vi "Step Add CONT W Parameters.vi"(0 "VISA resource name":refnum<visa-resource-name>, 1 "Continuity Test Paramameters":T2={"High Limit (0 - 10,000 ohms) (1000)"=1000.0, "Low Limit (0 - 10,000 ohms) (0)"=0.0, "Dwell Time (0.0, 0.4 - 999.9 seconds) (1.0)"=1.0, "Offset (0 - 10.00 ohms) (0)"=0.0, "Auto Offset (F: Off)"=FALSE} {"Offset (0 - 10.00 ohms) (0)" format="%.2f"; "Dwell Time (0.0, 0.4 - 999.9 seconds) (1.0)" format="%.1f"; "Low Limit (0 - 10,000 ohms) (0)" format="%.2f"; "High Limit (0 - 10,000 ohms) (1000)" format="%.2f"}, 2 "Internal Scanner Exists?":bool, 3 "Scanner Settings":T1={"Scan1"=1, "Scan2"=1, "Scan3"=1, "Scan4"=1, "Scan5"=1, "Scan6"=1, "Scan7"=1, "Scan8"=1, "Scan9"=1, "Scan10"=1, "Scan11"=1, "Scan12"=1, "Scan13"=1, "Scan14"=1, "Scan15"=1, "Scan16"=1} {"Scan16" scale=0.0..2.0; "Scan15" scale=0.0..2.0; "Scan14" scale=0.0..2.0; "Scan13" scale=0.0..2.0; "Scan12" scale=0.0..2.0; "Scan11" scale=0.0..2.0; "Scan10" scale=0.0..2.0; "Scan9" scale=0.0..2.0; "Scan8" scale=0.0..2.0; "Scan7" scale=0.0..2.0; "Scan6" scale=0.0..2.0; "Scan5" scale=0.0..2.0; "Scan4" scale=0.0..2.0; "Scan3" min=0 max=2 scale=0.0..2.0; "Scan2" min=0 max=2 scale=0.0..2.0; "Scan1" min=0 max=2 scale=0.0..2.0}, 7 "Step Selection (1-200)":i32=1, 9 "Add Step":bool, 11 "error in (no error)":errorcluster) -> (4 "VISA resource name out":refnum<visa-resource-name>, 15 "error out":errorcluster)   [LabVIEW 2012, in "Associated Research 78XX Series.lvlib"]
doc: "Sets the parameters for the CONT test mode for the given memory location."
uses:
  <instrlib>/Associated Research 78XX Series/Associated Research 78XX Series.lvlib
  <instrlib>/Associated Research 78XX Series/Public/Configure/Steps/Low Level/CONT Test Parameters.ctl
  <instrlib>/Associated Research 78XX Series/Public/Configure/Steps/Low Level/Scanner Settings.ctl
panel:
  # "Add"
  # "Edit"
  # "On\nOff"
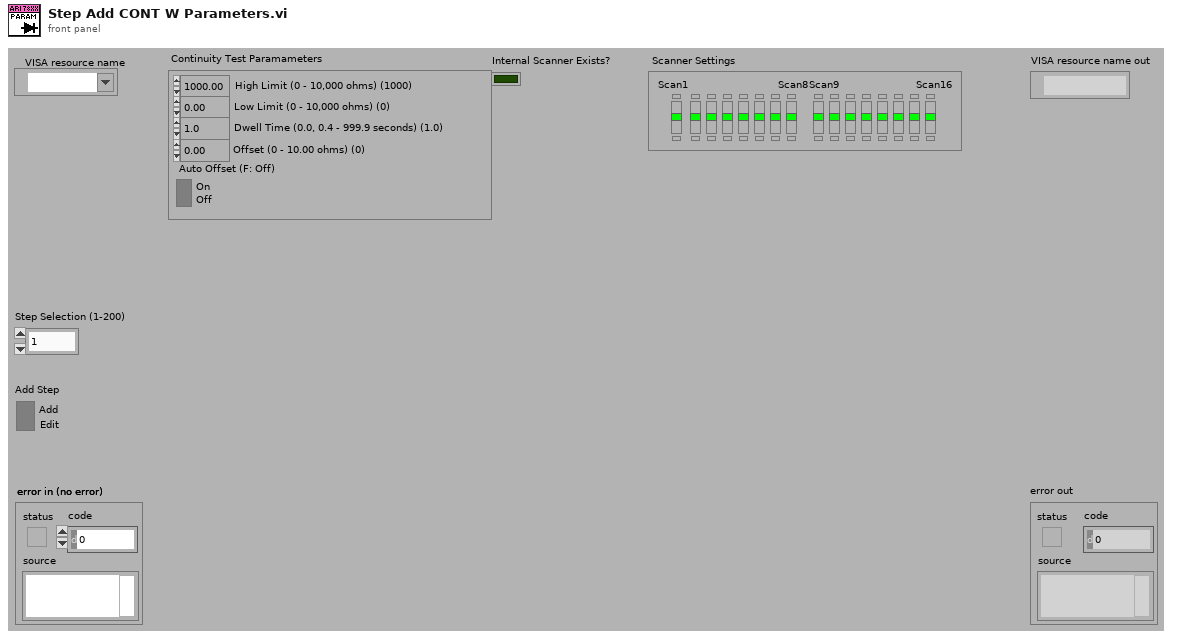
[diagram p1: front panel]
types:
  T1 = typedef "Associated Research 78XX Series.lvlib/Scanner Settings.ctl" = cluster{"Scan1":i32, "Scan2":i32, "Scan3":i32, "Scan4":i32, "Scan5":i32, "Scan6":i32, "Scan7":i32, "Scan8":i32, "Scan9":i32, "Scan10":i32, "Scan11":i32, "Scan12":i32, "Scan13":i32, "Scan14":i32, "Scan15":i32, "Scan16":i32}
  T2 = typedef "Associated Research 78XX Series.lvlib/CONT Test Parameters.ctl" = cluster{"High Limit (0 - 10,000 ohms) (1000)":dbl, "Low Limit (0 - 10,000 ohms) (0)":dbl, "Dwell Time (0.0, 0.4 - 999.9 seconds) (1.0)":dbl, "Offset (0 - 10.00 ohms) (0)":dbl, "Auto Offset (F: Off)":bool}
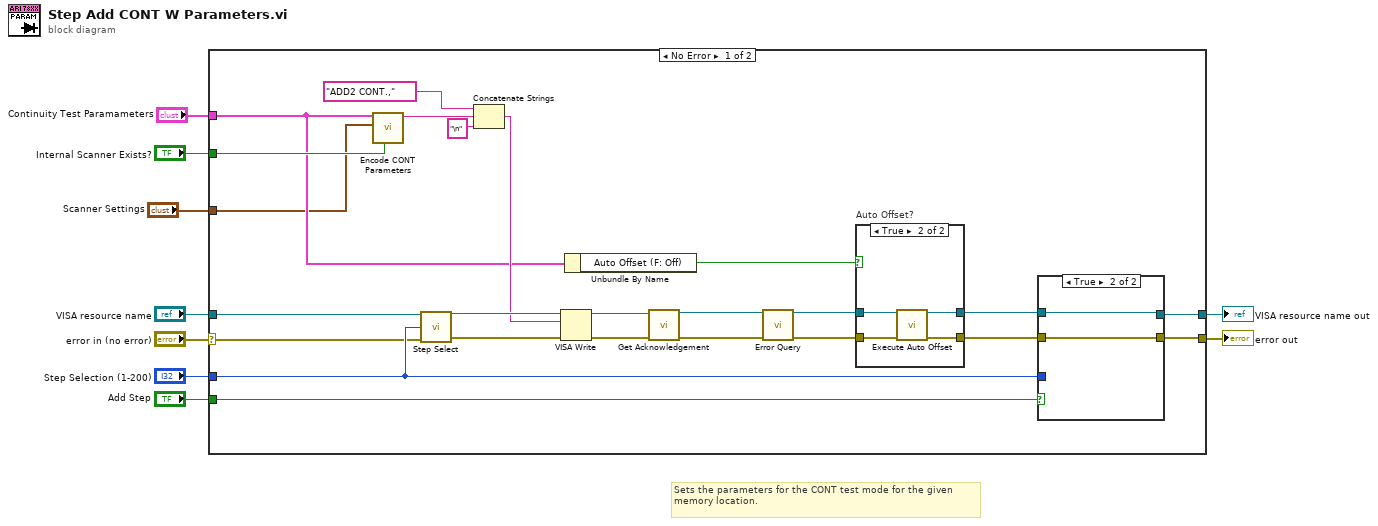
[diagram p0: block diagram]
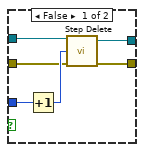
[diagram p3: hidden frame]
diagram:
  # "Sets the parameters for the CONT test mode for the given memory location."
  n1 = case shown="No Error" "error in (no error)" {
    selector: "error in (no error)" -> [w12 w49]
    tunnel: [w31 w49] -> w8
    tunnel: [w30 w48] -> w6
    tunnel: "VISA resource name" -> [w13 w48]
    tunnel: "Step Selection (1-200)" -> [w14 _]
    tunnel: "Add Step" -> [w29 _]
    tunnel: "Continuity Test Paramameters" -> [w16 _]
    tunnel: "Internal Scanner Exists?" -> [w28 _]
    tunnel: "Scanner Settings" -> [w15 _]
    frame No Error {
      n2 = call <instrlib>:"Encode CONT Parameters.vi"("Internal Scanner Exists?"=w28, "Scanner Settings"=w15, "Continuity Test Paramameters in"=w16) -> ("Add Step"=w27:string)  [unwired: 6 in, 2 out]
      n3 = call <instrlib>:"Step Select.vi"("VISA resource name"=w13, "Step Number (1)"=w14, "error in (no error)"=w12) -> ("VISA resource name out"=w32:refnum<visa-resource-name>, "error out"=w33:errorcluster)  [unwired: 11 in]
      n4 = Concatenate Strings("ADD2 CONT.," ("string"), w27, "\n" ("string")) -> (w25:string)
      n5 = VISA Write(VISA resource name=w32, write buffer=w25, error in (no error)=w33) -> (VISA resource name out=w11:refnum<visa-resource-name>, error out=w10:errorcluster)  [unwired: 1 out]
      n6 = Unbundle By Name(w16) -> ("Auto Offset (F: Off)"=w20:bool)
      n7 = call <instrlib>:"Get Acknowledgement.vi"("VISA resource name"=w11, "error in (no error)"=w10) -> ("VISA resource name out"=w19:refnum<visa-resource-name>, "error out"=w18:errorcluster)  [unwired: 12 in]
      n8 = call <instrlib>:"Error Query.vi"("VISA resource name"=w19, "error in (no error)"=w18) -> ("VISA resource name out"=w24:refnum<visa-resource-name>, "error out"=w23:errorcluster)  [unwired: 10 in, 2 out]
      n9 = case "Auto Offset?" shown="True" w20 {
        tunnel: w24 -> [w35 w39]
        tunnel: w23 -> [w34 w38]
        tunnel: [w34 w36] -> w22
        tunnel: [w35 w37] -> w21
        frame False {
        }
        frame True {
          n10 = call <instrlib>:"Execute Auto Offset.vi"("VISA resource name"=w39, "error in (no error)"=w38) -> ("VISA resource name out"=w37:refnum<visa-resource-name>, "error out"=w36:errorcluster)  [unwired: 12 in]
        }
      }
      n11 = case shown="True" w29 {
        tunnel: w14 -> [w45 _]
        tunnel: w22 -> [w43 w46]
        tunnel: w21 -> [w42 w47]
        tunnel: [w41 w46] -> w31
        tunnel: [w40 w47] -> w30
        frame False {
          n12 = Increment(x=w45) -> (x+1=w44:i32)
          n13 = call <instrlib>:"Step Delete.vi"("VISA resource name"=w42, "Step Number (0 = Active Step)"=w44, "error in (no error)"=w43) -> ("VISA resource name out"=w40:refnum<visa-resource-name>, "error out"=w41:errorcluster)  [unwired: 11 in]
        }
        frame True {
        }
      }
    }
    frame Error {
    }
  }
  "error out" <- w8
  "VISA resource name out" <- w6
